vi "Process_SetFlag.vi"(0 "ref in":T1, 1 "IndexArray":i32[](array[numeric]), 2 "FlagArray":bool[](array[boolean]), 3 "error in":errorcluster) -> (6 "ref out":T1, 9 "error out":errorcluster)   [LabVIEW 2015]
uses:
  Control/Process_Flag.ctl
panel:
  out "Timed out":bool
  in  "ms timeout (-1)":i32=-1
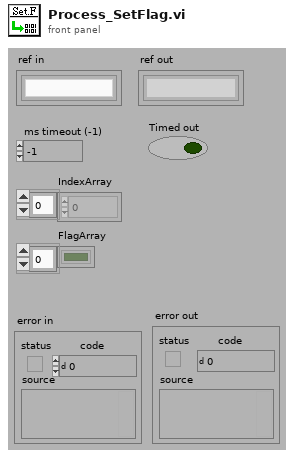
[diagram p1: front panel]
types:
  T1 = typedef "Error站_ref.ctl" = refnum<k1>
  T2 = typedef "Process_Flag.ctl" = cluster{"0":bool, "1":bool, "2":bool, "3":bool, "4":bool, "5":bool, "6":bool, "7":bool, "8":bool, "9":bool, "10":bool, "11":bool, "12":bool, "13":bool, "14":bool, "15":bool, "16":bool, "17":bool, "18":bool, "19":bool, "20":bool, "21":bool, "22":bool, "23":bool, "24":bool, "25":bool, "26":bool, "27":bool, "28":bool, "29":bool}
  T3 = enum16{"OpenReference", "CloseReference", "Get Data", "Set Data", "Set Flag"}
  T4 = typedef "Semaphore RefNum" = refnum<k1>
  T5 = cluster{"Flag out[0]":bool, "Flag out[1]":bool, "Flag out[2]":bool, "Flag out[3]":bool, "Flag out[4]":bool, "Flag out[5]":bool, "Flag out[6]":bool, "Flag out[7]":bool, "Flag out[8]":bool, "Flag out[9]":bool, "Flag out[10]":bool, "Flag out[11]":bool, "Flag out[12]":bool, "Flag out[13]":bool, "Flag out[14]":bool, "Flag out[15]":bool, "Flag out[16]":bool, "Flag out[17]":bool, "Flag out[18]":bool, "Flag out[19]":bool, "Flag out[20]":bool, "Flag out[21]":bool, "Flag out[22]":bool, "Flag out[23]":bool, "Flag out[24]":bool, "Flag out[25]":bool, "Flag out[26]":bool, "Flag out[27]":bool, "Flag out[28]":bool, "Flag out[29]":bool}
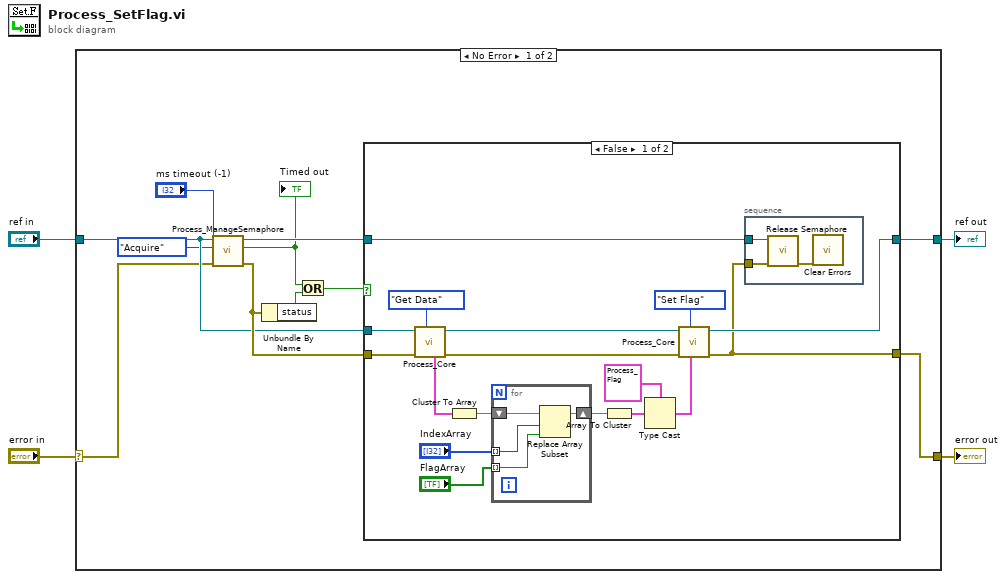
[diagram p0: block diagram]
diagram:
  n1 = case shown="No Error" "error in" {
    selector: "error in" -> [w6 w42]
    tunnel: [w10 w42] -> w3
    tunnel: "ref in" -> [w11 w41]
    tunnel: [w12 w41] -> w1
    frame No Error {
      n2 = call "Process_ManageSemaphore.vi"("error in (no error)"=w6, "ms timeout (-1)"="ms timeout (-1)", "Method (Acquire)"=enum8{"Acquire", "Destroy"}."Acquire", "ref"=w11) -> ("error out"=w15:errorcluster, "Timed out"=w7:bool, "semaphore out"=w13:T4)  [unwired: 1 in]
      "Timed out" <- w7
      n3 = Unbundle By Name(w15) -> ("status"=w8:bool)
      n4 = Or(x=w7, y=w8) -> (x .or. y?=w14:bool)
      n5 = case shown="False" w14 {
        tunnel: [w30 w39] -> w12
        tunnel: w13 -> [w31 _]
        tunnel: w15 -> [w28 w40]
        tunnel: [w29 w40] -> w10
        tunnel: w11 -> [w26 w39]
        frame False {
          n6 = call "Process_Core.vi"("Function"=T3."Get Data", "ref in"=w26) -> ("ref out"=w25:T1, "Flag out"=w23:T2)  [unwired: 6 in, 2 out]
          n7 = Cluster To Array(cluster=w23) -> (array=w22:bool[])
          n8 = for {
            shift-right: [w34] -> w21
            shift-left: w22 -> [w35]
            tunnel: "IndexArray" -> [w33] mode=indexing
            tunnel: "FlagArray" -> [w32] mode=indexing
            n9 = Replace Array Subset(array=w35, new element=w32, index=w33) -> (w34:bool[])
          }
          n10 = Array To Cluster(array=w21) -> (cluster=w17:T5)
          n11 = Type Cast(type=T2 {"0"=FALSE, "1"=FALSE, "2"=FALSE, "3"=FALSE, "4"=FALSE, "5"=FALSE, "6"=FALSE, "7"=FALSE, "8"=FALSE, "9"=FALSE, "10"=FALSE, "11"=FALSE, "12"=FALSE, "13"=FALSE, "14"=FALSE, "15"=FALSE, "16"=FALSE, "17"=FALSE, "18"=FALSE, "19"=FALSE, "20"=FALSE, "21"=FALSE, "22"=FALSE, "23"=FALSE, "24"=FALSE, "25"=FALSE, "26"=FALSE, "27"=FALSE, "28"=FALSE, "29"=FALSE} ("LoadTray_Flag"), x=w17) -> (*(type *) &x=w16:T2)
          n12 = call "Process_Core.vi"("Flag in"=w16, "Function"=T3."Set Flag", "error in"=w28, "ref in"=w25) -> ("error out"=w29:errorcluster, "ref out"=w30:T1)  [unwired: 4 in, 2 out]
          n13 = stacked-sequence {
            tunnel: w31 -> [w38]
            tunnel: w29 -> [w36]
            frame #0 {
              n14 = call <vilib>:"Release Semaphore.vi"("error in (no error)"=w36, "semaphore"=w38) -> ("error out"=w37:errorcluster)  [unwired: 4 in, 1 out]
              n15 = call <vilib>:"Clear Errors.vi"("error in (no error)"=w37) -> ()  [unwired: 5 in, 2 out]
            }
          }
        }
        frame True {
        }
      }
    }
    frame Error {
    }
  }
  "error out" <- w3
  "ref out" <- w1
